vi "FR Set TWM Measurement.vi"(4 "status ref (none)":refnum<vi>, 5 "Loop iteration":i32, 7 "Measurement properties":T1={"Measurement frequencies (Hz)"=[], "Sampling frequency (Hz)"=1.0, "Signal amplitude (V)"=50.0, "AC-DC settle time (s)"=50.0, "Record length (multiples of period)"=[], "Measurement template file"=path "", "Row of START keyword"=0, "Row of STOP keyword"=0, "Calculate RMS from samples"=FALSE, "AC-DC warm up time (s)"=300.0, "Measurement template line"=[], "DC meter readings No."=10, "Algorithm"="TWM-WFFT"} {"Record length (multiples of period)" format="%#_3p"; "Sampling frequency (Hz)" format="%#_3p"; "Measurement frequencies (Hz)" format="%#_3p"}, 8 "error in":errorcluster, 11 "handle":i32) -> (0 "error out":errorcluster, 3 "handle out":i32)   [LabVIEW 2020]
uses:
  Type definitions/FR Measuement properties.ctl
  external libraries/TWM-1.8.7.0-client/I64.vi
  external libraries/TWM-1.8.7.0-client/EXT.vi
  external libraries/TWM-1.8.7.0-client/String.vi
  external libraries/TWM-1.8.7.0-client/TWM Client.lvlib
  external libraries/TWM-1.8.7.0-client/infolib.lvlib
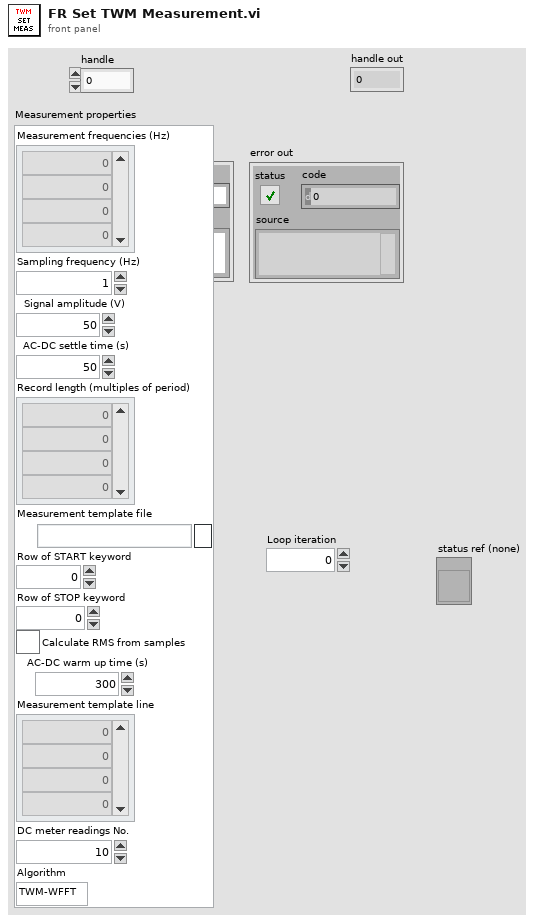
[diagram p1: front panel]
types:
  T1 = typedef "FR Measuement properties.ctl" = cluster{"Measurement frequencies (Hz)":dbl[], "Sampling frequency (Hz)":dbl, "Signal amplitude (V)":dbl, "AC-DC settle time (s)":dbl, "Record length (multiples of period)":dbl[], "Measurement template file":path, "Row of START keyword":i32, "Row of STOP keyword":i32, "Calculate RMS from samples":bool, "AC-DC warm up time (s)":dbl, "Measurement template line":i32[], "DC meter readings No.":i32, "Algorithm":string}
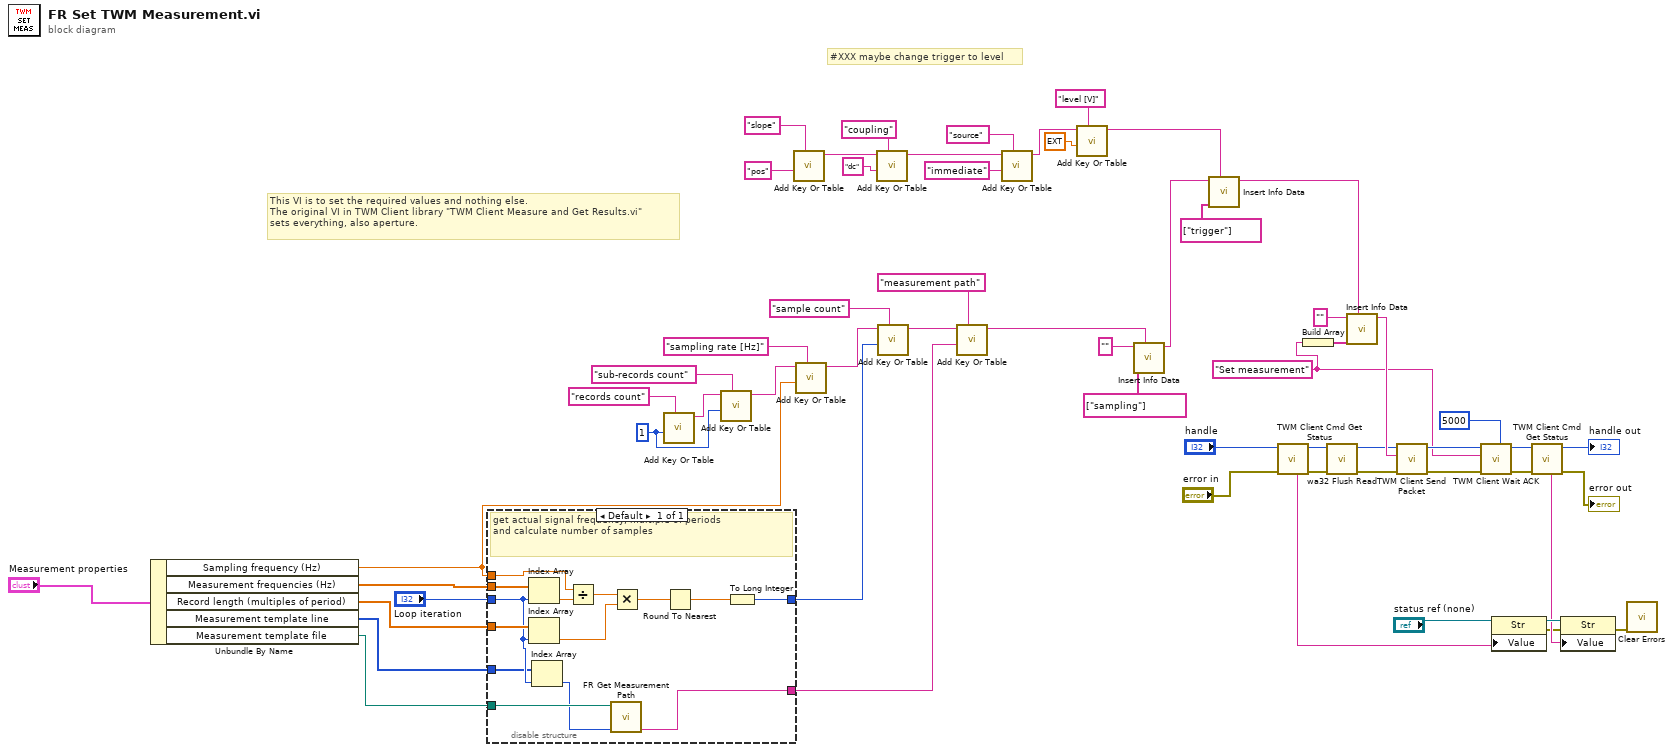
[diagram p0: block diagram]
diagram:
  w45 = 1 ("sub-records")
  w54 = "Set measurement" ("section name")
  # "#XXX maybe change trigger to level"
  # "This VI is to set the required values and nothing else.\nThe original VI in TWM Client library \"TWM Client Measure and Get Results.vi\"\nsets everything, also aperture."
  n1 = Unbundle By Name("Measurement properties") -> ("Sampling frequency (Hz)"=w8:dbl, "Measurement frequencies (Hz)"=w11:dbl[], "Record length (multiples of period)"=w10:dbl[], "Measurement template line"=w1:i32[], "Measurement template file"=w2:path)
  n2 = disable-structure shown="Default" {
    disable-tunnel: w11 -> [w74]
    disable-tunnel: w10 -> [w73]
    disable-tunnel: "Loop iteration" -> [w63]
    disable-tunnel: w8 -> [w72]
    disable-tunnel: [w66] -> w7
    disable-tunnel: [w65] -> w3
    disable-tunnel: w2 -> [w64]
    disable-tunnel: w1 -> [w62]
    frame Enabled {
      # "get actual signal frequency, multiple of periods\nand calculate number of samples"
      n3 = Index Array(array=w74, index=w63) -> (element=w71:dbl)
      n4 = Index Array(array=w73, index=w63) -> (element=w69:dbl)
      n5 = Index Array(array=w62, index=w63) -> (element=w61:i32)
      n6 = Divide(x=w72, y=w71) -> (x/y=w70:dbl)
      n7 = call "FR Get Measurement Path.vi"("Template line"=w61, "Measurement template file"=w64) -> ("Measurement path as string"=w65:string)  [unwired: 8 in, 1 out]
      n8 = Multiply(x=w70, y=w69) -> (x*y=w68:dbl)
      n9 = Round To Nearest(number=w68) -> (nearest integer value=w67:dbl)
      n10 = To Long Integer(number=w67) -> (32bit integer=w66:i32)
    }
  }
  n11 = call-poly "Add Key Or Table.vi"("key description"="records count", "numeric"=w45) -> ("info data out"=w48:string)  [unwired: 8 in, 1 out]
  n12 = call-poly "Add Key Or Table.vi"("key description"="sub-records count", "numeric"=w45, "info data"=w48) -> ("info data out"=w43:string)  [unwired: 7 in, 1 out]
  n13 = call-poly "Add Key Or Table.vi"("key description"="slope", "string"="pos" ("key description")) -> ("info data out"=w28:string)  [unwired: 8 in, 1 out]
  n14 = call-poly "Add Key Or Table.vi"("key description"="sampling rate [Hz]", "numeric"=w8, "info data"=w43) -> ("info data out"=w42:string)  [unwired: 7 in, 1 out]
  n15 = call-poly "Add Key Or Table.vi"("key description"="coupling", "string"="dc" ("key description"), "info data"=w28) -> ("info data out"=w32:string)  [unwired: 7 in, 1 out]
  n16 = call-poly "Add Key Or Table.vi"("key description"="sample count", "numeric"=w7, "info data"=w42) -> ("info data out"=w6:string)  [unwired: 7 in, 1 out]
  n17 = call-poly "Add Key Or Table.vi"("key description"="measurement path", "string"=w3, "info data"=w6) -> ("info data out"=w5:string)  [unwired: 7 in, 1 out]
  n18 = call-poly "Add Key Or Table.vi"("key description"="source", "string"="immediate" ("key description"), "info data"=w32) -> ("info data out"=w34:string)  [unwired: 7 in, 1 out]
  n19 = call-poly "Add Key Or Table.vi"("key description"="level [V]", "numeric"=ext 2.5, "info data"=w34) -> ("info data out"=w37:string)  [unwired: 7 in, 1 out]
  n20 = call "Insert Info Data.vi"("info data to insert"=w5, "sections"=string[] ["sampling"], "info data"="") -> ("info data out"=w41:string)  [unwired: 7 in, 1 out]
  n21 = call "Insert Info Data.vi"("info data to insert"=w37, "sections"=string[] ["trigger"], "info data"=w41) -> ("info data out"=w40:string)  [unwired: 7 in, 1 out]
  n22 = call "TWM Client Cmd Get Status.vi"("error in"="error in", "handle"="handle") -> ("error out"=w15:errorcluster, "handle out"=w26:i32, "status string"=w24:string)  [unwired: 5 in, 2 out]
  n23 = Build Array(w54) -> (w59:string[])
  n24 = call "wa32 Flush Read.vi"("error in"=w15, "handle"=w26) -> ("error out"=w53:errorcluster, "handle out"=w52:i32)  [unwired: 7 in, 1 out]
  n25 = call "Insert Info Data.vi"("info data to insert"=w40, "sections"=w59, "info data"="") -> ("info data out"=w60:string)  [unwired: 7 in, 1 out]
  n26 = call "TWM Client Send Packet.vi"("error in"=w53, "command string"=w60, "handle"=w52) -> ("error out"=w57:errorcluster, "handle out"=w56:i32)  [unwired: 7 in]
  n27 = call "TWM Client Wait ACK.vi"("timeout [ms] (3000)"=5000 ("timeout [ms] (1000)"), "error in"=w57, "command header"=w54, "handle"=w56) -> ("error out"=w22:errorcluster, "handle out"=w21:i32)  [unwired: 6 in]
  n28 = property class="Str"(reference="status ref (none)", "Value"=w24) -> (reference out=w23:refnum<vi>, error out=w16:errorcluster)  [unwired: 1 in]
  n29 = call "TWM Client Cmd Get Status.vi"("error in"=w22, "handle"=w21) -> ("error out"=→"error out":errorcluster, "handle out"=→"handle out":i32, "status string"=w18:string)  [unwired: 5 in, 2 out]
  n30 = property class="Str"(reference=w23, error in=w16, "Value"=w18) -> (error out=w17:errorcluster)  [unwired: 1 out]
  n31 = call <vilib>:"Clear Errors.vi"("error in (no error)"=w17) -> ()  [unwired: 5 in, 2 out]
